vi "GrabFrame.vi"(8 "error in (no error)":errorcluster, 10 "Image":u16[][](array[numeric]), 11 "InterferometrUI in":refnum<class "InterferometerUI.lvclass">) -> (0 "error out":errorcluster, 3 "InterferometrUI out":refnum<class "InterferometerUI.lvclass">)   [LabVIEW 2023, in "InterferometrUI.lvlib" / "InterferometerUI.lvclass"]
uses:
  InterferometerUI.lvclass
  InterferometerUI.lvclass/InterferometerUI.ctl
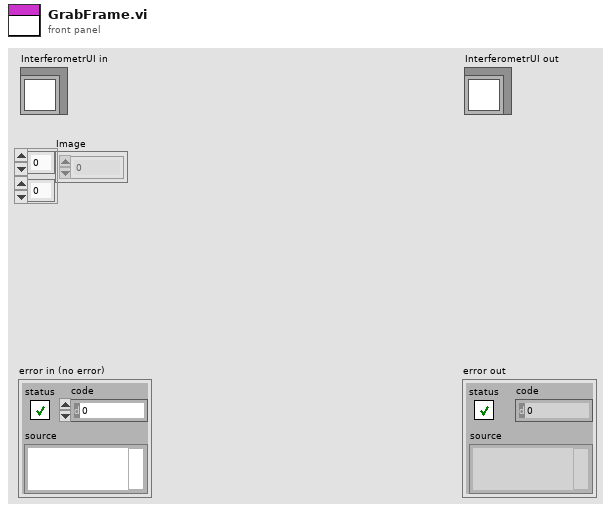
[diagram p1: front panel]
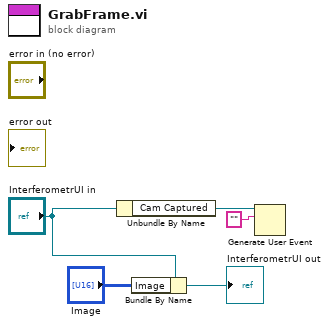
[diagram p0: block diagram]
diagram:
  n1 = Unbundle By Name("InterferometrUI in") -> ("Cam Captured"=w5:refnum<user-event>)
  n2 = Bundle By Name(cluster="InterferometrUI in", "Image"="Image") -> (→"InterferometrUI out":refnum<class "InterferometerUI.lvclass">)
  n3 = Generate User Event(user event=w5, event data cluster="" ("event data")) -> ()  [unwired: 2 in, 2 out]
